vi "Read Target Time.vi"(8 "error in (no error)":errorcluster, 11 "TimerSensorConfig in":refnum<class "TimerSensorConfig.lvclass">) -> (0 "error out":errorcluster, 2 "Target Time":timestamp, 3 "TimerSensorConfig out":refnum<class "TimerSensorConfig.lvclass">)   [LabVIEW 2012, in "TimerSensor.lvlib" / "TimerSensorConfig.lvclass"]
uses:
  TimerSensorConfig.lvclass
  TimerSensorConfig.lvclass/TimerSensorConfig.ctl
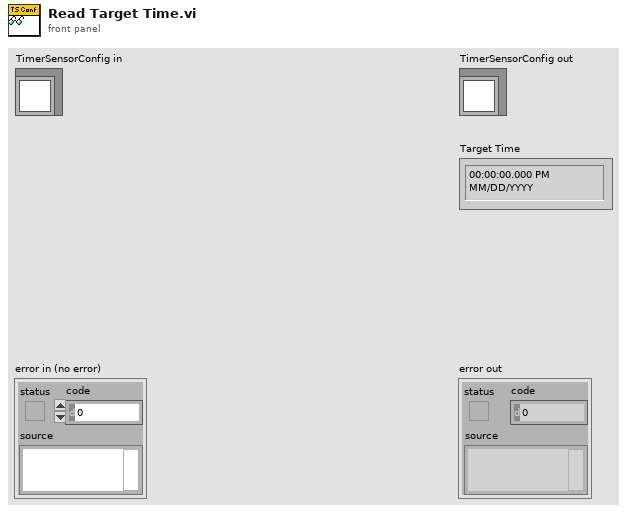
[diagram p1: front panel]
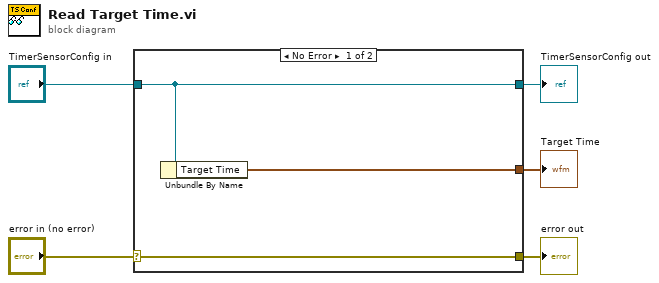
[diagram p0: block diagram]
diagram:
  n1 = case shown="No Error" "error in (no error)" {
    selector: "error in (no error)" -> [w8 w9]
    tunnel: [w8 w9] -> w4
    tunnel: [w7 w10] -> w2
    tunnel: "TimerSensorConfig in" -> [w7 w10]
    tunnel: [w6 _] -> w1
    frame No Error {
      n2 = Unbundle By Name(w7) -> ("Target Time"=w6:timestamp)
    }
    frame Error {
    }
  }
  "error out" <- w4
  "TimerSensorConfig out" <- w2
  "Target Time" <- w1
